vi "SetStrikeoutFont__slk_tc.vi"(0 "tree control in":refnum<class "TreeControl.lvclass">, 5 "input tag (current tag)":string, 11 "error in (no error)":errorcluster, 12 "column # (entire row=-2)":i32=-2) -> (4 "tree control out":refnum<class "TreeControl.lvclass">, 6 "output tag":string, 15 "error out":errorcluster)   [LabVIEW 2020, in "TreeControl.lvclass"]
doc: "Sets the font to STRIKEOUT of input tag with specified column."
uses:
  Library/TreeControl.lvclass
  Library/TreeControl.lvclass/TreeControl.ctl
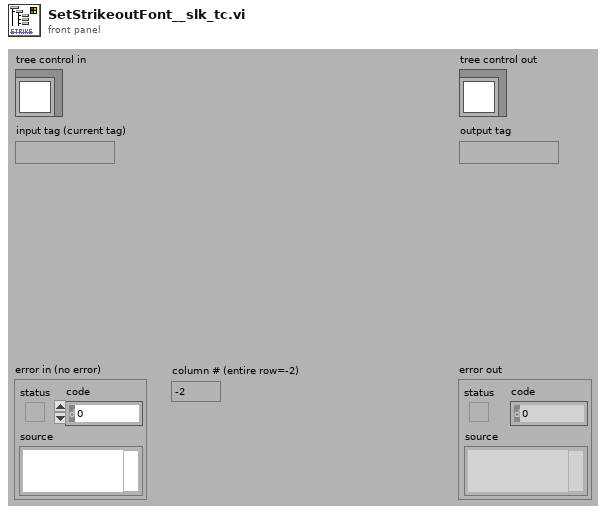
[diagram p1: front panel]
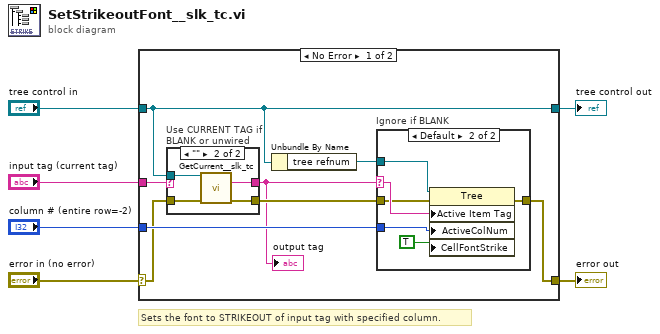
[diagram p0: block diagram]
diagram:
  # "Sets the font to STRIKEOUT of input tag with specified column."
  n1 = case shown="No Error" "error in (no error)" {
    selector: "error in (no error)" -> [w9 w29]
    tunnel: [w8 w29] -> w5
    tunnel: [w13 w28] -> w3
    tunnel: "tree control in" -> [w13 w28]
    tunnel: "input tag (current tag)" -> [w14 _]
    tunnel: "column # (entire row=-2)" -> [w11 _]
    frame No Error {
      n2 = case "Use CURRENT TAG if BLANK or unwired" shown="\"\"" w14 {
        selector: w14 -> [w23 _]
        tunnel: [w23 w27] -> w7
        tunnel: w13 -> [_ w26]
        tunnel: w9 -> [w22 w25]
        tunnel: [w22 w24] -> w10
        frame Default {
        }
        frame "" {
          n3 = call "GetCurrent__slk_tc.vi"("tree control in"=w26, "error in (no error)"=w25) -> ("current tag"=w27:string, "error out"=w24:errorcluster)  [unwired: 1 in, 11 out]
        }
      }
      "output tag" <- w7
      n4 = Unbundle By Name(w13) -> ("tree refnum"=w12:refnum<vi>)
      n5 = case "Ignore if BLANK" shown="Default" w7 {
        selector: w7 -> [_ w20]
        tunnel: w12 -> [_ w21]
        tunnel: w11 -> [_ w19]
        tunnel: w10 -> [w15 w17]
        tunnel: [w15 w16] -> w8
        frame "" {
        }
        frame Default {
          n6 = property class="Tree"(reference=w21, error in=w17, "Active Item Tag"=w20, "ActiveColNum"=w19, "CellFontStrike"=TRUE ("Active Cell:Cell Font:Bold")) -> (error out=w16:errorcluster)  [unwired: 1 out]
        }
      }
    }
    frame Error {
    }
  }
  "error out" <- w5
  "tree control out" <- w3
